vi "tale of three indices -- check state.vi"(6 "query":T2, 11 "tale of three indices":T3={"left"=0, "center"=0, "right"=0, "right most"=0, "left most"=0, "window"=0, "max win factor"=2, "max win"=2, "min win"=2}) -> (1 "balance state":T1(ring), 2 "answer":bool)   [LabVIEW 2018]
uses:
  tale of three indices -- int -- control.ctl
  tale of three indices --state.ctl
  Q - not nan -- integer.vi
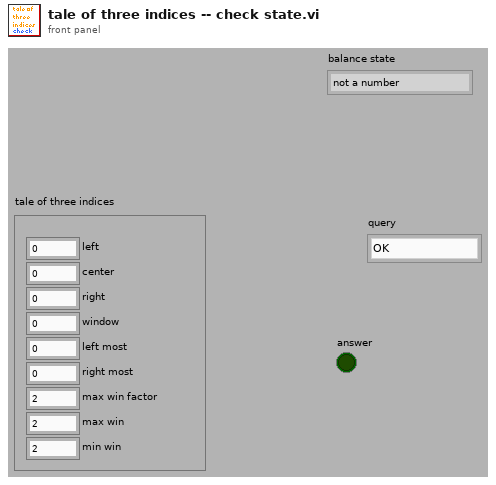
[diagram p1: front panel]
types:
  T1 = enum16{"not a number", "above", "in range", "below"}
  T2 = typedef "tale of three indices --state.ctl" = enum16{"OK", "window stuck at left", "window stuck at right", "left wing shrink - able", "right wing shrink- able", "left wing broaden - able", "window right - able", "right wing broaden - able", "window left - able", "broaden - able", "shrink - able", "center right - able", "center left - able", "balance state"}
  T3 = typedef "tale of three indices -- int -- control.ctl" = cluster{"left":i32, "center":i32, "right":i32, "right most":i32, "left most":i32, "window":i32, "max win factor":i32, "max win":i32, "min win":i32}
  T4 = typedef "comparison control.ctl" = enum16{"not a number", "above", "in range", "below"}
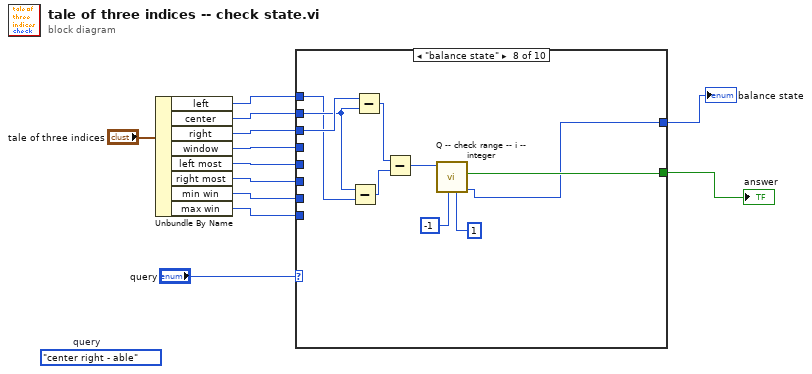
[diagram p0: block diagram]
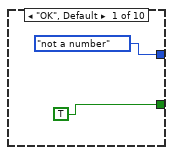
[diagram p2: hidden frame]
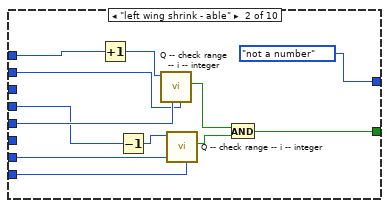
[diagram p3: hidden frame]
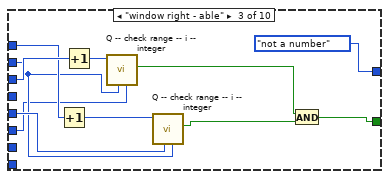
[diagram p4: hidden frame]
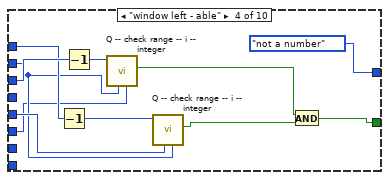
[diagram p5: hidden frame]
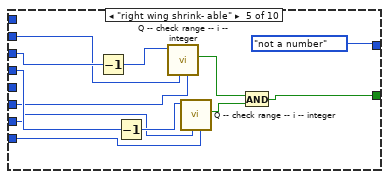
[diagram p6: hidden frame]
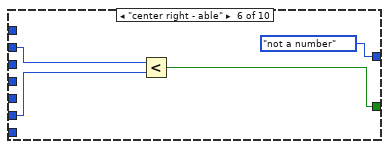
[diagram p7: hidden frame]
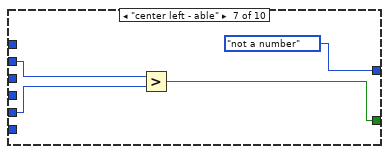
[diagram p8: hidden frame]
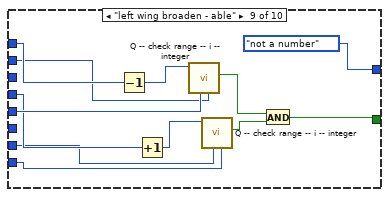
[diagram p9: hidden frame]
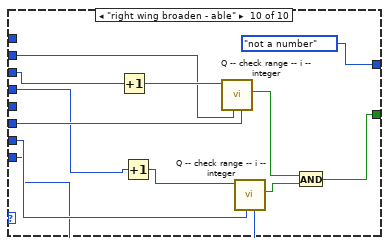
[diagram p10: hidden frame]
diagram:
  (unwired) tale_of_three_indices_--state."center right - able"  # query
  n1 = Unbundle By Name("tale of three indices") -> ("left"=w10:i32, "center"=w8:i32, "right"=w2:i32, "window"=w7:i32, "left most"=w9:i32, "right most"=w3:i32, "min win"=w6:i32, "max win"=w5:i32)
  n2 = case shown="\"balance state\"" "query" {
    tunnel: w10 -> [_ w24 w32 w43 _ _ _ w71 w86 _]
    tunnel: w9 -> [_ w22 w31 w42 _ _ w66 _ w85 _]
    tunnel: w8 -> [_ w21 w30 w41 w51 w64 w68 w72 w84 w98]
    tunnel: w7 -> [_ w20 _ _ w56 _ _ _ w83 w96]
    tunnel: w6 -> [_ w18 _ _ w54 _ _ _ w81 w94]
    tunnel: w5 -> [_ w17 _ _ w53 _ _ _ w80 w93]
    tunnel: [TRUE w16 w28 w39 w52 w62 w67 w70 w87 w92] -> w4
    tunnel: w3 -> [_ _ w29 w40 w50 w63 _ _ _ w97]
    tunnel: w2 -> [_ _ w33 w44 w57 _ _ w73 _ w99]
    tunnel: [T1."not a number" ("selector") T1."not a number" ("selector") T1."not a number" ("selector") T1."not a number" ("selector") T1."not a number" ("selector") T1."not a number" ("selector") T1."not a number" ("selector") w69 T1."not a number" ("selector") T1."not a number" ("selector")] -> w1
    frame "OK", Default {
    }
    frame "left wing shrink - able" {
      n3 = Increment(x=w24) -> (x+1=w23:i32)
      n4 = Decrement(x=w20) -> (x-1=w19:i32)
      n5 = call "Q -- check range -- i -- integer.vi"("upper"=w21, "lower"=w22, "number"=w23) -> ("in range?"=w25:bool)  [unwired: 6 in, 2 out]
      n6 = call "Q -- check range -- i -- integer.vi"("upper"=w17, "lower"=w18, "number"=w19) -> ("in range?"=w26:bool)  [unwired: 6 in, 2 out]
      n7 = And(x=w25, y=w26) -> (x .and. y?=w16:bool)
    }
    frame "window right - able" {
      n8 = Increment(x=w32) -> (x+1=w36:i32)
      n9 = Increment(x=w33) -> (x+1=w37:i32)
      n10 = call "Q -- check range -- i -- integer.vi"("upper"=w29, "lower"=w30, "number"=w37) -> ("in range?"=w35:bool)  [unwired: 6 in, 2 out]
      n11 = call "Q -- check range -- i -- integer.vi"("upper"=w30, "lower"=w31, "number"=w36) -> ("in range?"=w34:bool)  [unwired: 6 in, 2 out]
      n12 = And(x=w35, y=w34) -> (x .and. y?=w28:bool)
    }
    frame "window left - able" {
      n13 = Decrement(x=w43) -> (x-1=w47:i32)
      n14 = Decrement(x=w44) -> (x-1=w48:i32)
      n15 = call "Q -- check range -- i -- integer.vi"("upper"=w40, "lower"=w41, "number"=w48) -> ("in range?"=w46:bool)  [unwired: 6 in, 2 out]
      n16 = call "Q -- check range -- i -- integer.vi"("upper"=w41, "lower"=w42, "number"=w47) -> ("in range?"=w45:bool)  [unwired: 6 in, 2 out]
      n17 = And(x=w46, y=w45) -> (x .and. y?=w39:bool)
    }
    frame "right wing shrink- able" {
      n18 = Decrement(x=w57) -> (x-1=w60:i32)
      n19 = Decrement(x=w56) -> (x-1=w55:i32)
      n20 = call "Q -- check range -- i -- integer.vi"("upper"=w50, "lower"=w51, "number"=w60) -> ("in range?"=w58:bool)  [unwired: 6 in, 2 out]
      n21 = call "Q -- check range -- i -- integer.vi"("upper"=w53, "lower"=w54, "number"=w55) -> ("in range?"=w59:bool)  [unwired: 6 in, 2 out]
      n22 = And(x=w58, y=w59) -> (x .and. y?=w52:bool)
    }
    frame "center right - able" {
      n23 = Less?(x=w64, y=w63) -> (x < y?=w62:bool)
    }
    frame "center left - able" {
      n24 = Greater?(x=w68, y=w66) -> (0:w67:bool)
    }
    frame "balance state" {
      n25 = Subtract(x=w72, y=w71) -> (x-y=w77:i32)
      n26 = Subtract(x=w73, y=w72) -> (x-y=w78:i32)
      n27 = Subtract(x=w78, y=w77) -> (x-y=w76:i32)
      n28 = call "Q -- check range -- i -- integer.vi"("upper"=1, "lower"=-1, "number"=w76) -> ("selector"=w69:T4, "in range?"=w70:bool)  [unwired: 6 in, 1 out]
    }
    frame "left wing broaden - able" {
      n29 = Decrement(x=w86) -> (x-1=w90:i32)
      n30 = Increment(x=w83) -> (x+1=w82:i32)
      n31 = call "Q -- check range -- i -- integer.vi"("upper"=w84, "lower"=w85, "number"=w90) -> ("in range?"=w88:bool)  [unwired: 6 in, 2 out]
      n32 = call "Q -- check range -- i -- integer.vi"("upper"=w80, "lower"=w81, "number"=w82) -> ("in range?"=w89:bool)  [unwired: 6 in, 2 out]
      n33 = And(x=w88, y=w89) -> (x .and. y?=w87:bool)
    }
    frame "right wing broaden - able" {
      n34 = Increment(x=w99) -> (x+1=w102:i32)
      n35 = Increment(x=w96) -> (x+1=w95:i32)
      n36 = call "Q -- check range -- i -- integer.vi"("upper"=w97, "lower"=w98, "number"=w102) -> ("in range?"=w100:bool)  [unwired: 6 in, 2 out]
      n37 = call "Q -- check range -- i -- integer.vi"("upper"=w93, "lower"=w94, "number"=w95) -> ("in range?"=w101:bool)  [unwired: 6 in, 2 out]
      n38 = And(x=w100, y=w101) -> (x .and. y?=w92:bool)
    }
  }
  "answer" <- w4
  "balance state" <- w1
